vi "BuildCustomDashBoardData.vi"   [LabVIEW 2013]
doc: "This VI builds data and sends it back to the dashboard PC program. By default it sends back the raw values for the first analog, digital, and solenoid module. Modify it to send back the data you want to view. Consider adding higher level data to the Dashboard Datatype.ctl and to this VI. Then update the Dashboard to display the data however you like.\n\nThis software is licensed. Open the labview\\readme\\WPI Robotics Library Open Source License.txt file for more information."
uses:
  <vilib>/Rock Robotics/WPI/DriverStation/WPI_DriverStationDigitalData.ctl
  typedefs/Dashboard Datatype.ctl
  typedefs/DashboardEnable.ctl
  typedefs/custom dash data.ctl
  typedefs/subStates.ctl
  typedefs/vision data.ctl
  <vilib>/Rock Robotics/WPI/Joystick/WPI_JoystickButtonState.ctl
  typedefs/fg_typedef.ctl
  <vilib>/Rock Robotics/SystemInterfaces/System/FPGA_SystemGet.vi
  <vilib>/Rock Robotics/WPI/Joystick/WPI_JoystickGetSetRefNum.vi
  <vilib>/NI_Real-Time Target Support.lvlib
types:
  T1 = typedef "custom dash data.ctl" = cluster{"Motors":cluster{"Pickup Motor":dbl, "Pickup Belt":dbl, "Pickup Distance ":dbl, "Pickup Rate":dbl, "Right Motor":dbl, "Left Motor":dbl}, "substates":cluster{"Latch":T2, "Pickup Arm":T2, "Belts":T2, "Shooter":T2, "Drive":T2}, "Safeties":cluster{"Arm Safety":bool, "Arm Limit":bool}, "Performance":cluster{"CPU Usage":dbl, "Vision mSPI":u32, "Main mSPI":u32}, "Data":T3, "Joysticks":cluster{"J1 Axes":cluster{"axis 1 (x)":dbl, "axis 2 (y)":dbl, "axis 3 (throttle)":dbl, "axis 4":dbl, "axis 5":dbl, "axis 6":dbl}, "J1 Buttons":T4, "J2 Axes":cluster{"axis 1 (x)":dbl, "axis 2 (y)":dbl, "axis 3 (throttle)":dbl, "axis 4":dbl, "axis 5":dbl, "axis 6":dbl}, "J2 Buttons":T4, "J3 Axes":cluster{"axis 1 (x)":dbl, "axis 2 (y)":dbl, "axis 3 (throttle)":dbl, "axis 4":dbl, "axis 5":dbl, "axis 6":dbl}, "J3 Buttons":T4}, "SubSystem Manager":cluster{"Ball State Read":enum16{"no ball", "holding", "loaded"}, "Picked Up":bool, "Loaded":bool, "Shooter Cocked":bool, "Arm Ready":bool}, "Vision Enabled?":bool}
  T2 = typedef "subStates.ctl" = enum16{"null", "wait", "driver control", "auto", "manual override", "hold position", "rotate", "pickup", "pass", "load", "goto shoot", "shoot", "cancel", "end"}
  T3 = typedef "vision data.ctl" = cluster{"x":dbl, "y":dbl, "area":dbl, "width":dbl, "height":dbl, "Hot Goal Present?":bool, "distance":dbl}
  T4 = typedef "WPI_JoystickButtonState.ctl" = cluster{"Button 1":bool, "Button 2":bool, "Button 3":bool, "Button 4":bool, "Button 5":bool, "Button 6":bool, "Button 7":bool, "Button 8":bool, "Button 9":bool, "Button 10":bool, "Button 11":bool, "Button 12":bool}
  T5 = typedef "DashboardEnable.ctl" = cluster{"Analog Module 1":bool[], "Analog Module 2":bool[], "Digital Module 1":bool, "Digital Module 2":bool, "Solenoid Module":bool}
  T6 = typedef "Dashboard Datatype.ctl" = cluster{cluster{"AnalogModule[0]":cluster{"Channel[0]":sgl, "Channel[1]":sgl, "Channel[2]":sgl, "Channel[3]":sgl, "Channel[4]":sgl, "Channel[5]":sgl, "Channel[6]":sgl, "Channel[7]":sgl}, "AnalogModule[1]":cluster{"Channel[0]":sgl, "Channel[1]":sgl, "Channel[2]":sgl, "Channel[3]":sgl, "Channel[4]":sgl, "Channel[5]":sgl, "Channel[6]":sgl, "Channel[7]":sgl}}, cluster{"DigitalModule[0]":T7, "DigitalModule[1]":T7}, "Solenoid":u8}
  T7 = typedef "WPI_DriverStationDigitalData.ctl" = cluster{"Relay Fwd":u8, "Relay Rev":u8, "GPIO":u16, "GPIO_OE":u16, "PWM":cluster{"PWM[0]":u8, "PWM[1]":u8, "PWM[2]":u8, "PWM[3]":u8, "PWM[4]":u8, "PWM[5]":u8, "PWM[6]":u8, "PWM[7]":u8, "PWM[8]":u8, "PWM[9]":u8}}
  T8 = typedef "fg_typedef.ctl" = enum16{"Get", "Set"}
  T9 = cluster{"AnalogModule[0]":cluster{"Channel[0]":sgl, "Channel[1]":sgl, "Channel[2]":sgl, "Channel[3]":sgl, "Channel[4]":sgl, "Channel[5]":sgl, "Channel[6]":sgl, "Channel[7]":sgl}, "AnalogModule[1]":cluster{"Channel[0]":sgl, "Channel[1]":sgl, "Channel[2]":sgl, "Channel[3]":sgl, "Channel[4]":sgl, "Channel[5]":sgl, "Channel[6]":sgl, "Channel[7]":sgl}}
  T10 = cluster{"DigitalModule[0]":T7, "DigitalModule[1]":T7}
  T11 = cluster{"Channel[0]":sgl, "Channel[1]":sgl, "Channel[2]":sgl, "Channel[3]":sgl, "Channel[4]":sgl, "Channel[5]":sgl, "Channel[6]":sgl, "Channel[7]":sgl}[]
  T12 = cluster{"Channel[0]":sgl, "Channel[1]":sgl, "Channel[2]":sgl, "Channel[3]":sgl, "Channel[4]":sgl, "Channel[5]":sgl, "Channel[6]":sgl, "Channel[7]":sgl}
  T13 = cluster{"AnalogModule[0][0]":sgl, "AnalogModule[0][1]":sgl, "AnalogModule[0][2]":sgl, "AnalogModule[0][3]":sgl, "AnalogModule[0][4]":sgl, "AnalogModule[0][5]":sgl, "AnalogModule[0][6]":sgl, "AnalogModule[0][7]":sgl}
  T14 = cluster{"[0]":cluster{"Channel[0]":sgl, "Channel[1]":sgl, "Channel[2]":sgl, "Channel[3]":sgl, "Channel[4]":sgl, "Channel[5]":sgl, "Channel[6]":sgl, "Channel[7]":sgl}, "[1]":cluster{"Channel[0]":sgl, "Channel[1]":sgl, "Channel[2]":sgl, "Channel[3]":sgl, "Channel[4]":sgl, "Channel[5]":sgl, "Channel[6]":sgl, "Channel[7]":sgl}}
  T15 = typedef "FPGA_DIODevRef.ctl" = cluster{"DevStatus":errorcluster, "Module":T16}
  T16 = typedef "FPGA_TypedefDigitalModule.ctl" = enum16{"Digital Module 1", "Digital Module 2"}
  T17 = cluster{"[0]":u8, "[1]":u8, "[2]":u8, "[3]":u8, "[4]":u8, "[5]":u8, "[6]":u8, "[7]":u8, "[8]":u8, "[9]":u8}
  T18 = typedef "FPGA_SolenoidDevRef.ctl" = cluster{"DevStatus":errorcluster, "Module":T19}
  T19 = typedef "FPGA_TypedefSolenoidModule.ctl" = enum16{"Solenoid Module 1", "Solenoid Module 2"}
  T20 = cluster{"Pickup Motor":dbl, "Pickup Belt":dbl, "Pickup Distance ":dbl, "Pickup Rate":dbl, "Right Motor":dbl, "Left Motor":dbl}
  T21 = cluster{"CPU Usage":dbl, "Vision mSPI":u32, "Main mSPI":u32}
  T22 = typedef "WPI_EncoderDevRef.ctl" = cluster{"DevStatus":errorcluster, "EncoderIndex":T23, "CounterIndex":T24, "DistancePerCount":dbl, "Decoding Type":T25}
  T23 = typedef "FPGA_EncoderIdx.ctl" = enum8{"Enc 0", "Enc 1", "Enc 2", "Enc 3", "Invalid"}
  T24 = typedef "FPGA_CounterCtrSystemIndex.ctl" = enum8{"Ctr 0", "Ctr 1", "Ctr 2", "Ctr 3", "Ctr 4", "Ctr 5", "Ctr 6", "Ctr 7", "Invalid"}
  T25 = typedef "WPI_EncoderType.ctl" = enum16{"1x", "2x", "4x"}
  T26 = typedef "WPI_MotorControlDeviceRef.ctl" = cluster{"DeviceStatus":errorcluster, "Type":enum16{"PWM", "CAN"}, "PWM":cluster{"Digital Module":T16, "PWM Channel":T27, "DeadBand":T28}, "CAN":cluster{"Device Number":u8, "Control Mode":T29, "Semaphore":T30, "Max Vout":dbl}, "Invert":bool, "TransformRef":T31, "InvTransformRef":T31}
  T27 = typedef "FPGA_DIOPWMChannel.ctl" = enum8{"PWM 1", "PWM 2", "PWM 3", "PWM 4", "PWM 5", "PWM 6", "PWM 7", "PWM 8", "PWM 9", "PWM 10", "Invalid"}
  T28 = typedef "WPI_PWMDeadband.ctl" = cluster{"Name":string, "maxPositivePwm":i32, "minPositivePwm":i32, "centerPwm":i32, "maxNegativePwm":i32, "minNegativePwm":i32, "angularRange":u16}
  T29 = typedef "WPI_CANJaguar_ControlMode.ctl" = enum8{"Percent VBus", "Current", "Speed", "Position", "Voltage"}
  T30 = typedef "Semaphore RefNum" = refnum<k1>
  T31 = typedef "WPI_PWMTransform_ConPane.ctl" = refnum<vi>
  T32 = typedef "NI_Real-Time Target Support.lvlib/RT CPU Load.ctl" = cluster{"Total (%)":dbl, "Time Critical (%)":dbl, "Timed Structures (%)":dbl, "High (%)":dbl, "Above Normal (%)":dbl, "Normal (%)":dbl, "Background (%)":dbl, "Idle (%)":dbl, "ISR (%)":dbl}
  T33 = cluster{"Vision mSPI":u32, "Main mSPI":u32, "Dash mSPI":u32}
  T34 = cluster{"Ball State Read":enum16{"no ball", "holding", "loaded"}, "Picked Up":bool, "Loaded":bool, "Shooter Cocked":bool, "Arm Ready":bool}
  T35 = typedef "WPI_JoystickDevRef.ctl" = cluster{"Device":T36}
  T36 = typedef "WPI_JoystickDeviceEnum.ctl" = enum16{"USB 1", "USB 2", "USB 3", "USB 4", "Kinect 1", "Kinect 2"}
  T37 = cluster{"axis 1 (x)":dbl, "axis 2 (y)":dbl, "axis 3 (throttle)":dbl, "axis 4":dbl, "axis 5":dbl, "axis 6":dbl}
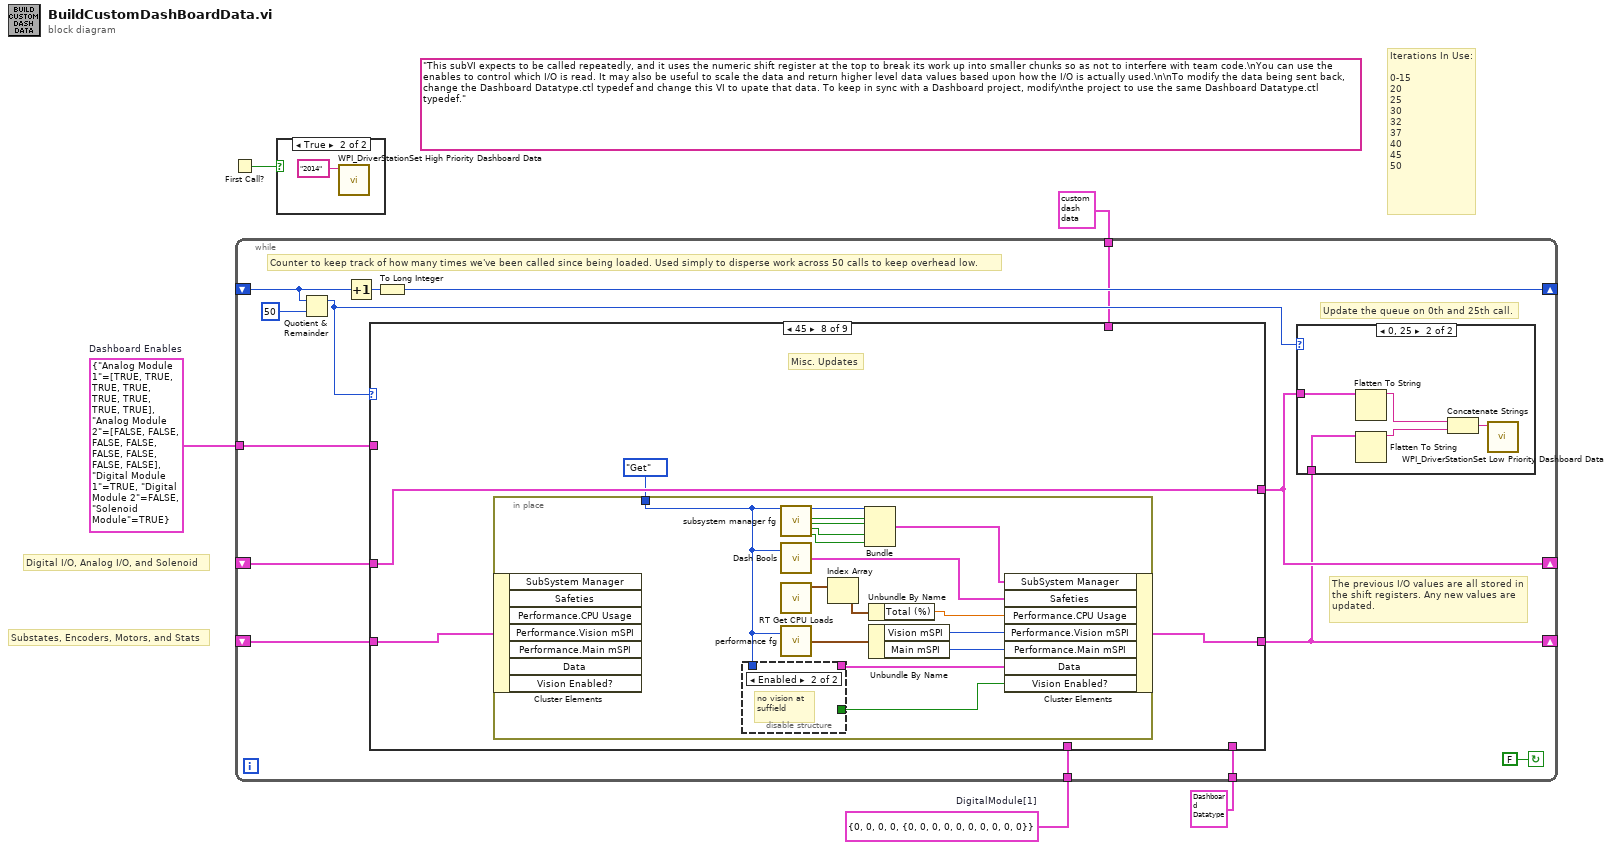
[diagram p0: block diagram]
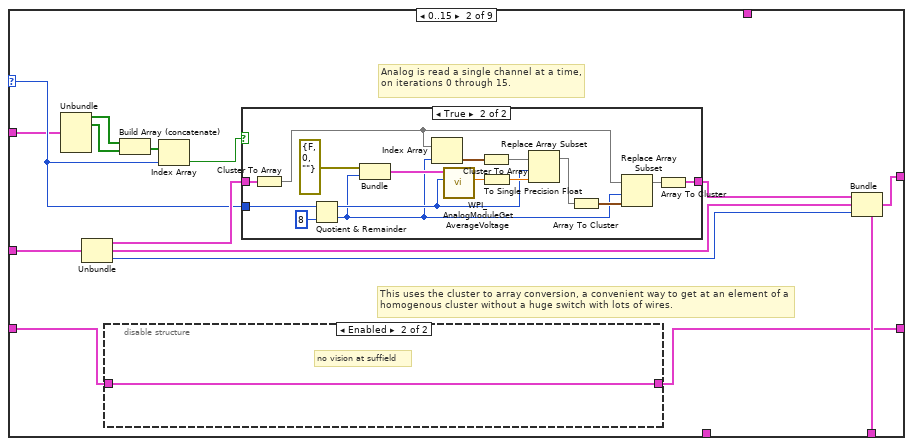
[diagram p5: hidden frame]
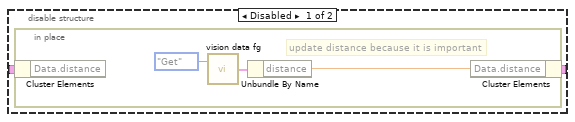
[diagram p6: hidden frame]
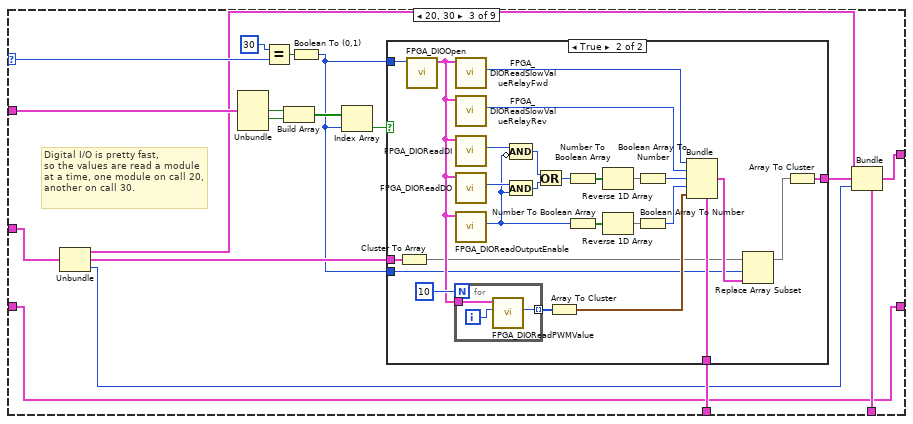
[diagram p8: hidden frame]
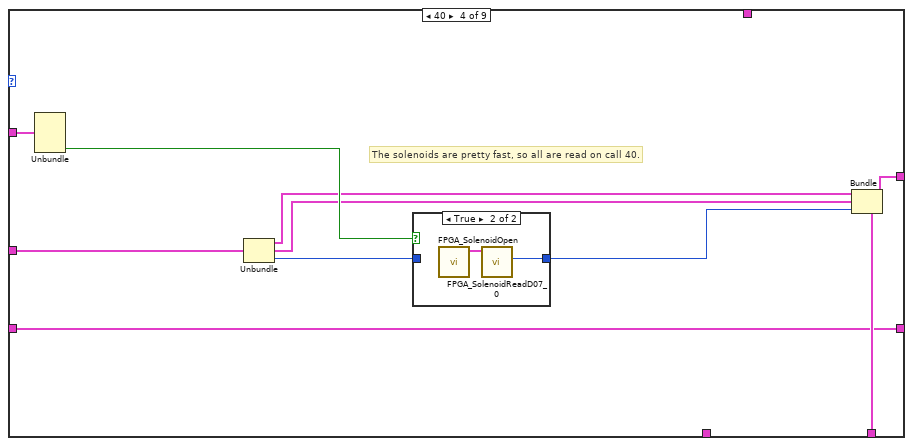
[diagram p10: hidden frame]
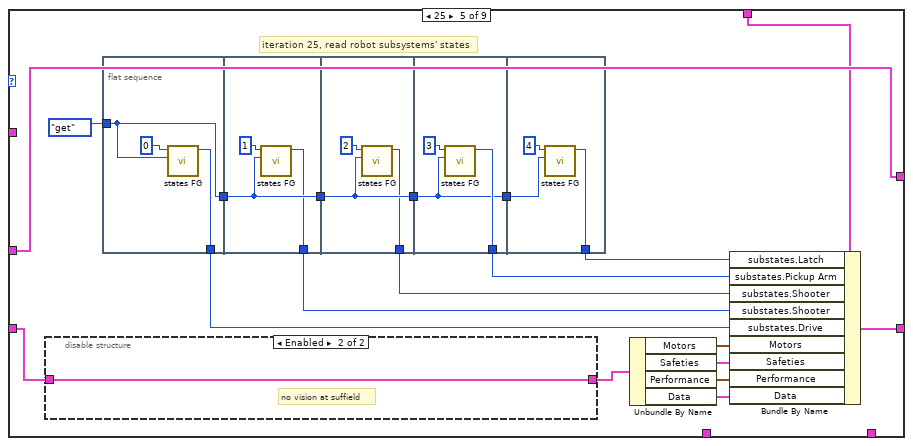
[diagram p12: hidden frame]
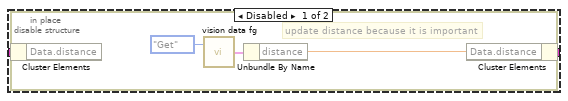
[diagram p13: hidden frame]
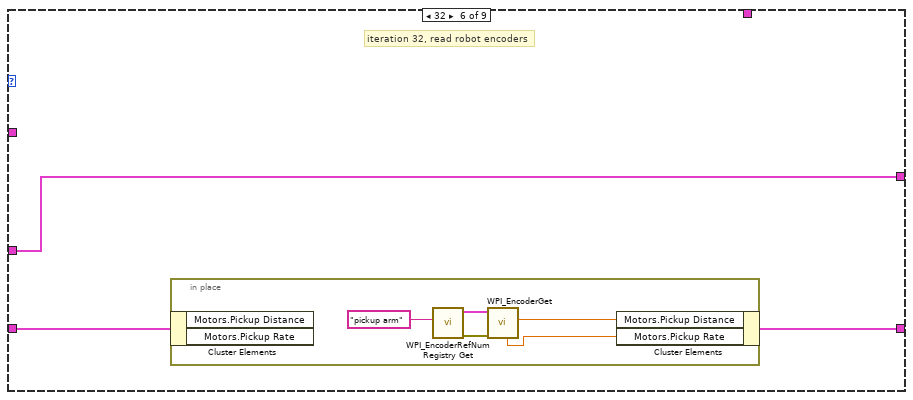
[diagram p14: hidden frame]
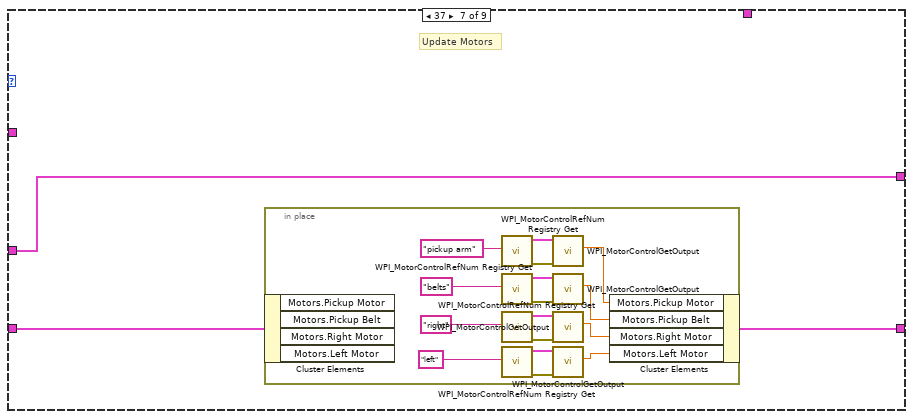
[diagram p15: hidden frame]
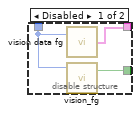
[diagram p16: hidden frame]
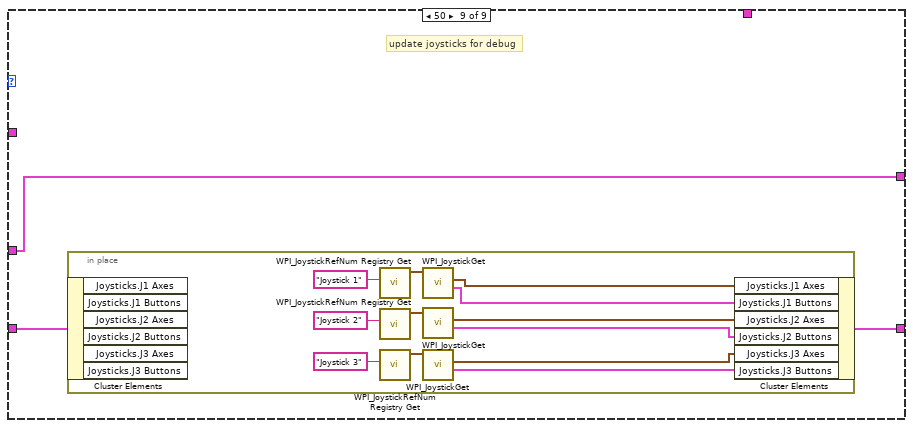
[diagram p17: hidden frame]
diagram:
  w5 = T5 {"Analog Module 1"=[TRUE, TRUE, TRUE, TRUE, TRUE, TRUE, TRUE, TRUE], "Analog Module 2"=[FALSE, FALSE, FALSE, FALSE, FALSE, FALSE, FALSE, FALSE], "Digital Module 1"=TRUE, "Digital Module 2"=FALSE, "Solenoid Module"=TRUE}  # Dashboard Enables
  (unwired) "This subVI expects to be called repeatedly, and it uses the numeric shift register at the top to break its work up into smaller chunks so as not to interfere with team code.\nYou can use the enables to control which I/O is read. It may also be useful to scale the data and return higher level data values based upon how the I/O is actually used.\n\nTo modify the data being sent back, change the Dashboard Datatype.ctl typedef and change this VI to upate that data. To keep in sync with a Dashboard project, modify\nthe project to use the same Dashboard Datatype.ctl typedef."
  w4 = T7 {"Relay Fwd"=0, "Relay Rev"=0, "GPIO"=0, "GPIO_OE"=0, "PWM"={"PWM[0]"=0, "PWM[1]"=0, "PWM[2]"=0, "PWM[3]"=0, "PWM[4]"=0, "PWM[5]"=0, "PWM[6]"=0, "PWM[7]"=0, "PWM[8]"=0, "PWM[9]"=0}}  # DigitalModule[1]
  # "Iterations In Use:\n\n0-15\n20\n25\n30\n32\n37\n40\n45\n50"
  # "Substates, Encoders, Motors, and Stats"
  # "Digital I/O, Analog I/O, and Solenoid"
  n1 = First Call?() -> (First Call?: T/F=w3:bool)
  n2 = while {
    shift-right: [w12] -> _
    shift-left: _ -> [w14]
    shift-right: [w9] -> _
    shift-left: _ -> [w17]
    tunnel: w4 -> [w16]
    tunnel: T6 {{"AnalogModule[0]"={"Channel[0]"=0.0, "Channel[1]"=0.0, "Channel[2]"=0.0, "Channel[3]"=0.0, "Channel[4]"=0.0, "Channel[5]"=0.0, "Channel[6]"=0.0, "Channel[7]"=0.0}, "AnalogModule[1]"={"Channel[0]"=0.0, "Channel[1]"=0.0, "Channel[2]"=0.0, "Channel[3]"=0.0, "Channel[4]"=0.0, "Channel[5]"=0.0, "Channel[6]"=0.0, "Channel[7]"=0.0}}, {"DigitalModule[0]"={"Relay Fwd"=0, "Relay Rev"=0, "GPIO"=0, "GPIO_OE"=0, "PWM"={"PWM[0]"=0, "PWM[1]"=0, "PWM[2]"=0, "PWM[3]"=0, "PWM[4]"=0, "PWM[5]"=0, "PWM[6]"=0, "PWM[7]"=0, "PWM[8]"=0, "PWM[9]"=0}}, "DigitalModule[1]"={"Relay Fwd"=0, "Relay Rev"=0, "GPIO"=0, "GPIO_OE"=0, "PWM"={"PWM[0]"=0, "PWM[1]"=0, "PWM[2]"=0, "PWM[3]"=0, "PWM[4]"=0, "PWM[5]"=0, "PWM[6]"=0, "PWM[7]"=0, "PWM[8]"=0, "PWM[9]"=0}}}, "Solenoid"=0} ("Dashboard Data") -> [w11]
    tunnel: w5 -> [w10]
    shift-right: [w6] -> _
    shift-left: _ -> [w7]
    tunnel: T1 {"Motors"={"Pickup Motor"=0.0, "Pickup Belt"=0.0, "Pickup Distance "=0.0, "Pickup Rate"=0.0, "Right Motor"=0.0, "Left Motor"=0.0}, "substates"={"Latch"=enum."null", "Pickup Arm"=enum."null", "Belts"=enum."null", "Shooter"=enum."null", "Drive"=enum."null"}, "Safeties"={"Arm Safety"=FALSE, "Arm Limit"=FALSE}, "Performance"={"CPU Usage"=0.0, "Vision mSPI"=0, "Main mSPI"=0}, "Data"={"x"=0.0, "y"=0.0, "area"=0.0, "width"=0.0, "height"=0.0, "Hot Goal Present?"=FALSE, "distance"=0.0}, "Joysticks"={"J1 Axes"={"axis 1 (x)"=0.0, "axis 2 (y)"=0.0, "axis 3 (throttle)"=0.0, "axis 4"=0.0, "axis 5"=0.0, "axis 6"=0.0}, "J1 Buttons"={"Button 1"=FALSE, "Button 2"=FALSE, "Button 3"=FALSE, "Button 4"=FALSE, "Button 5"=FALSE, "Button 6"=FALSE, "Button 7"=FALSE, "Button 8"=FALSE, "Button 9"=FALSE, "Button 10"=FALSE, "Button 11"=FALSE, "Button 12"=FALSE}, "J2 Axes"={"axis 1 (x)"=0.0, "axis 2 (y)"=0.0, "axis 3 (throttle)"=0.0, "axis 4"=0.0, "axis 5"=0.0, "axis 6"=0.0}, "J2 Buttons"={"Button 1"=FALSE, "Button 2"=FALSE, "Button 3"=FALSE, "Button 4"=FALSE, "Button 5"=FALSE, "Button 6"=FALSE, "Button 7"=FALSE, "Button 8"=FALSE, "Button 9"=FALSE, "Button 10"=FALSE, "Button 11"=FALSE, "Button 12"=FALSE}, "J3 Axes"={"axis 1 (x)"=0.0, "axis 2 (y)"=0.0, "axis 3 (throttle)"=0.0, "axis 4"=0.0, "axis 5"=0.0, "axis 6"=0.0}, "J3 Buttons"={"Button 1"=FALSE, "Button 2"=FALSE, "Button 3"=FALSE, "Button 4"=FALSE, "Button 5"=FALSE, "Button 6"=FALSE, "Button 7"=FALSE, "Button 8"=FALSE, "Button 9"=FALSE, "Button 10"=FALSE, "Button 11"=FALSE, "Button 12"=FALSE}}, "SubSystem Manager"={"Ball State Read"=enum."no ball", "Picked Up"=FALSE, "Loaded"=FALSE, "Shooter Cocked"=FALSE, "Arm Ready"=FALSE}, "Vision Enabled?"=FALSE} ("Custom Dash Data") -> [w8]
    stop <- FALSE continue-if-true
    # "Counter to keep track of how many times we've been called since being loaded. Used simply to disperse work across 50 calls to keep overhead low."
    # "Update the queue on 0th and 25th call."
    # "The previous I/O values are all stored in\nthe shift registers. Any new values are\nupdated."
    n3 = Quotient & Remainder(x=w14, y=50) -> (x-y*floor(x/y)=w13:i32)  [unwired: 1 out]
    n4 = Increment(x=w14) -> (x+1=w19:i32)
    n5 = case shown="45" w13 {
      selector: w13 -> [_ w36 w78 _ _ _ _ _ _]
      tunnel: [w26 w32 w69 w119 w134 w167 w176 w195 w218] -> w9
      tunnel: w17 -> [w26 w31 w71 w121 w134 w167 w176 w195 w218]
      tunnel: w16 -> [_ _ w82 _ _ _ _ _ _]
      tunnel: w11 -> [_ w38 w70 w118 _ _ _ _ _]
      tunnel: w10 -> [_ w35 w76 w122 _ _ _ _ _]
      tunnel: w8 -> [_ _ _ _ w132 _ _ _ _]
      tunnel: [w25 w27 w67 w115 w133 w168 w175 w196 w216] -> w6
      tunnel: w7 -> [w25 w28 w67 w115 w128 w166 w174 w194 w217]
      frame Default {
        # "Don't update any I/O"
      }
      frame 0..15 {
        # "This uses the cluster to array conversion, a convenient way to get at an element of a\nhomogenous cluster without a huge switch with lots of wires."
        # "Analog is read a single channel at a time,\non iterations 0 through 15."
        n6 = Unbundle(w35) -> ("Analog Module 1"=w34:bool[], "Analog Module 2"=w33:bool[])  [unwired: 3 out]
        n7 = Unbundle(w31) -> (w37:T9, w30:T10, "Solenoid"=w29:u8)
        n8 = disable-structure shown="Enabled" {
          disable-tunnel: w28 -> [w43 w47]
          disable-tunnel: [w42 w47] -> w27
          frame Disabled {
            n9 = in-place {
              # "update distance because it is important"
              n10 = in-place-cluster #1(w43) -> ()  [unwired: 1 out]
              n11 = call "vision data fg.vi"("Menu"=fg_typedef."Get") -> ("Output"=w45:T3)  [unwired: 1 in]
              n12 = Unbundle By Name(w45) -> ("distance"=w44:dbl)
              n13 = in-place-cluster #1("Data.distance"=w44) -> (w42:T1)
            }
          }
          frame Enabled {
            # "no vision at suffield"
          }
        }
        n14 = Build Array (concatenate)(w34, w33) -> (w40:bool[])
        n15 = Index Array(array=w40, index=w36) -> (element=w41:bool)
        n16 = case shown="True" w41 {
          tunnel: w36 -> [_ w55]
          tunnel: [w48 w52] -> w39
          tunnel: w37 -> [w48 w51]
          frame False {
          }
          frame True {
            n17 = Cluster To Array(cluster=w51) -> (array=w50:T11)
            n18 = Quotient & Remainder(x=w55, y=8) -> (x-y*floor(x/y)=w54:i32, floor(x/y)=w49:i32)
            n19 = Bundle("DevStatus"=errorcluster {"status"=FALSE, "code"=0, "source"=""}, w49) -> (w63:cluster{"DevStatus":errorcluster, i32})  [unwired: 1 out]
            n20 = Index Array(array=w50, index=w49) -> (element=w57:T12)
            n21 = call <vilib>:"WPI_AnalogModuleGetAverageVoltage.vi"("Channel"=w54, "AnalogModuleDevStatus"=w63) -> ("Average Voltage"=w60:dbl)  [unwired: 1 in, 8 out]
            n22 = Cluster To Array(cluster=w57) -> (array=w56:sgl[])
            n23 = To Single Precision Float(number=w60) -> (single precision float=w59:sgl)
            n24 = Replace Array Subset(array=w56, new element=w59, index=w54) -> (w58:sgl[])
            n25 = Array To Cluster(array=w58) -> (cluster=w62:T13)
            n26 = Replace Array Subset(array=w50, new element=w62, index=w49) -> (w53:T11)
            n27 = Array To Cluster(array=w53) -> (cluster=w52:T14)
          }
        }
        n28 = Bundle(cluster=w38, w39, w30, "Solenoid"=w29) -> (w32:T6)
      }
      frame 20, 30 {
        # "Digital I/O is pretty fast,\nso the values are read a module\nat a time, one module on call 20,\nanother on call 30."
        n29 = Unbundle(w71) -> (w66:T9, w73:T10, "Solenoid"=w65:u8)
        n30 = Unbundle(w76) -> ("Digital Module 1"=w75:bool, "Digital Module 2"=w74:bool)  [unwired: 3 out]
        n31 = Equal?(x=30, y=w78) -> (x = y?=w80:bool)
        n32 = Build Array(w75, w74) -> (w77:bool[])
        n33 = Boolean To (0,1)(Boolean=w80) -> (0, 1=w68:i16)
        n34 = Index Array(array=w77, index=w68) -> (element=w79:bool)
        n35 = case shown="True" w79 {
          tunnel: w82 -> [_ w91]
          tunnel: [w83 w84] -> w72
          tunnel: w68 -> [_ w89]
          tunnel: w68 -> [_ w88]
          tunnel: w73 -> [w83 w87]
          frame False {
          }
          frame True {
            n36 = Cluster To Array(cluster=w87) -> (array=w86:T7[])
            n37 = call <vilib>:"FPGA_DIOOpen.vi"("Module (Module 1)"=w89) -> ("DIODeviceRef"=w107:T15)  [unwired: 1 in, 9 out]
            n38 = for {
              N: 10 -> [_]
              tunnel: w107 -> [w112]
              tunnel: [w110] -> w108 mode=indexing
              i -> [w111]
              n39 = call <vilib>:"FPGA_DIOReadPWMValue.vi"("PWMChannel"=w111, "DIODeviceRef In"=w112) -> ("PWMValue"=w110:u8)  [unwired: 1 in, 8 out]
            }
            n40 = call <vilib>:"FPGA_DIOReadSlowValueRelayFwd.vi"("DIODeviceRef In"=w107) -> ("Relay Forward"=w100:u8)  [unwired: 1 in, 9 out]
            n41 = call <vilib>:"FPGA_DIOReadSlowValueRelayRev.vi"("DIODeviceRef In"=w107) -> ("Relay Reverse"=w101:u8)  [unwired: 1 in, 9 out]
            n42 = call <vilib>:"FPGA_DIOReadDI.vi"("DIODeviceRef In"=w107) -> ("DI"=w105:u16)  [unwired: 1 in, 9 out]
            n43 = call <vilib>:"FPGA_DIOReadDO.vi"("DIODeviceRef In"=w107) -> ("DO"=w104:u16)  [unwired: 1 in, 9 out]
            n44 = call <vilib>:"FPGA_DIOReadOutputEnable.vi"("DIODeviceRef In"=w107) -> ("OutputEnable"=w95:u16)  [unwired: 1 in, 9 out]
            n45 = And(x=w104, y=w95) -> (x .and. y?=w103:u16)
            n46 = Compound Arithmetic op=AND(w105, invert w95) -> (w102:u16)
            n47 = Or(x=w102, y=w103) -> (x .or. y?=w93:u16)
            n48 = Array To Cluster(array=w108) -> (cluster=w106:T17)
            n49 = Number To Boolean Array(number=w93) -> (Boolean array=w98:bool[])
            n50 = Number To Boolean Array(number=w95) -> (Boolean array=w97:bool[])
            n51 = Reverse 1D Array(array=w98) -> (reversed array=w99:bool[])
            n52 = Reverse 1D Array(array=w97) -> (reversed array=w96:bool[])
            n53 = Boolean Array To Number(Boolean array=w99) -> (number=w92:u32)
            n54 = Boolean Array To Number(Boolean array=w96) -> (number=w94:u32)
            n55 = Bundle(cluster=w91, "Relay Fwd"=w100, "Relay Rev"=w101, "GPIO"=w92, "GPIO_OE"=w94, "PWM"=w106) -> (w90:T7)
            n56 = Replace Array Subset(array=w86, new element=w90, index=w88) -> (w85:T7[])
            n57 = Array To Cluster(array=w85) -> (cluster=w84:cluster{"[0]":T7, "[1]":T7})
          }
        }
        n58 = Bundle(cluster=w70, w66, w72, "Solenoid"=w65) -> (w69:T6)
      }
      frame 40 {
        # "The solenoids are pretty fast, so all are read on call 40."
        n59 = Unbundle(w122) -> ("Solenoid Module"=w116:bool)  [unwired: 4 out]
        n60 = Unbundle(w121) -> (w114:T9, w113:T10, "Solenoid"=w120:u8)
        n61 = case shown="True" w116 {
          tunnel: [w123 w124] -> w117
          tunnel: w120 -> [w123 _]
          frame False {
          }
          frame True {
            n62 = call <vilib>:"FPGA_SolenoidOpen.vi"() -> ("SolenoidDevRef"=w125:T18)  [unwired: 2 in, 9 out]
            n63 = call <vilib>:"FPGA_SolenoidReadD07_0.vi"("SolenoidDevRef"=w125) -> ("DO7:0"=w124:u8)  [unwired: 1 in, 9 out]
          }
        }
        n64 = Bundle(cluster=w118, w114, w113, "Solenoid"=w117) -> (w119:T6)
      }
      frame 25 {
        # "iteration 25, read robot subsystems' states"
        n65 = disable-structure shown="Enabled" {
          disable-tunnel: w128 -> [w146 w150]
          disable-tunnel: [w145 w150] -> w127
          frame Disabled {
            n66 = in-place {
              # "update distance because it is important"
              n67 = in-place-cluster #2(w146) -> ()  [unwired: 1 out]
              n68 = call "vision data fg.vi"("Menu"=fg_typedef."Get") -> ("Output"=w148:T3)  [unwired: 1 in]
              n69 = Unbundle By Name(w148) -> ("distance"=w147:dbl)
              n70 = in-place-cluster #2("Data.distance"=w147) -> (w145:T1)
            }
          }
          frame Enabled {
            # "no vision at suffield"
          }
        }
        n71 = flat-sequence {
          tunnel: enum16{"set", "get"}."get" ("menu (get)") -> [w153]
          tunnel: [w153] -> w141
          tunnel: [w151] -> w135
          tunnel: [w156] -> w142
          tunnel: w141 -> [w156]
          tunnel: [w154] -> w136
          tunnel: [w159] -> w143
          tunnel: w142 -> [w159]
          tunnel: [w157] -> w137
          tunnel: w143 -> [w160]
          tunnel: [w161] -> w138
          tunnel: [w160] -> w140
          tunnel: w140 -> [w164]
          tunnel: [w163] -> w139
          frame #0 {
            n72 = call "states FG.vi"("menu (get)"=w153, "Loop ID"=0) -> ("subState out"=w151:T2)  [unwired: 6 in, 3 out]
          }
          frame #1 {
            n73 = call "states FG.vi"("menu (get)"=w156, "Loop ID"=1) -> ("subState out"=w154:T2)  [unwired: 6 in, 3 out]
          }
          frame #2 {
            n74 = call "states FG.vi"("menu (get)"=w159, "Loop ID"=2) -> ("subState out"=w157:T2)  [unwired: 6 in, 3 out]
          }
          frame #3 {
            n75 = call "states FG.vi"("menu (get)"=w160, "Loop ID"=3) -> ("subState out"=w161:T2)  [unwired: 6 in, 3 out]
          }
          frame #4 {
            n76 = call "states FG.vi"("menu (get)"=w164, "Loop ID"=4) -> ("subState out"=w163:T2)  [unwired: 6 in, 3 out]
          }
        }
        n77 = Unbundle By Name(w127) -> ("Motors"=w126:T20, "Safeties"=w131:cluster{"Arm Safety":bool, "Arm Limit":bool}, "Performance"=w130:T21, "Data"=w129:T3)
        n78 = Bundle By Name(cluster=w132, "substates.Latch"=w139, "substates.Pickup Arm"=w138, "substates.Shooter"=w137, "substates.Shooter"=w136, "substates.Drive"=w135, "Motors"=w126, "Safeties"=w131, "Performance"=w130, "Data"=w129) -> (w133:T1)
      }
      frame 32 {
        # "iteration 32, read robot encoders"
        n79 = in-place {
          n80 = in-place-cluster #3(w166) -> ()  [unwired: 2 out]
          n81 = call <vilib>:"WPI_EncoderRefNum Registry Get.vi"("refnum name"="pickup arm") -> ("error out"=w172:errorcluster, "EncoderDevRef"=w173:T22)  [unwired: 9 in]
          n82 = call <vilib>:"WPI_EncoderGet.vi"("error in (no error)"=w172, "EncoderDevRef"=w173) -> ("Distance"=w170:dbl, "Rate"=w169:dbl)  [unwired: 4 in, 4 out]
          n83 = in-place-cluster #3("Motors.Pickup Distance"=w170, "Motors.Pickup Rate"=w169) -> (w168:T1)
        }
      }
      frame 37 {
        # "Update Motors"
        n84 = in-place {
          n85 = in-place-cluster #4(w174) -> ()  [unwired: 4 out]
          n86 = call <vilib>:"WPI_MotorControlRefNum Registry Get.vi"("refnum name"="pickup arm") -> ("error out"=w185:errorcluster, "MotorControlDevRef"=w189:T26)  [unwired: 9 in]
          n87 = call <vilib>:"WPI_MotorControlRefNum Registry Get.vi"("refnum name"="belts") -> ("error out"=w186:errorcluster, "MotorControlDevRef"=w192:T26)  [unwired: 9 in]
          n88 = call <vilib>:"WPI_MotorControlRefNum Registry Get.vi"("refnum name"="right") -> ("error out"=w184:errorcluster, "MotorControlDevRef"=w182:T26)  [unwired: 9 in]
          n89 = call <vilib>:"WPI_MotorControlRefNum Registry Get.vi"("refnum name"="left") -> ("error out"=w179:errorcluster, "MotorControlDevRef"=w181:T26)  [unwired: 9 in]
          n90 = call <vilib>:"WPI_MotorControlGetOutput.vi"("error in (no error)"=w185, "MotorControlDevRef"=w189) -> ("Output"=w188:dbl)  [unwired: 7 in, 2 out]
          n91 = call <vilib>:"WPI_MotorControlGetOutput.vi"("error in (no error)"=w186, "MotorControlDevRef"=w192) -> ("Output"=w187:dbl)  [unwired: 7 in, 2 out]
          n92 = call <vilib>:"WPI_MotorControlGetOutput.vi"("error in (no error)"=w184, "MotorControlDevRef"=w182) -> ("Output"=w177:dbl)  [unwired: 7 in, 2 out]
          n93 = call <vilib>:"WPI_MotorControlGetOutput.vi"("error in (no error)"=w179, "MotorControlDevRef"=w181) -> ("Output"=w178:dbl)  [unwired: 7 in, 2 out]
          n94 = in-place-cluster #4("Motors.Pickup Motor"=w188, "Motors.Pickup Belt"=w187, "Motors.Right Motor"=w177, "Motors.Left Motor"=w178) -> (w175:T1)
        }
      }
      frame 45 {
        # "Misc. Updates"
        n95 = in-place {
          in-place-border: fg_typedef."Get" ("Menu (Get)") -> [w198]
          n96 = in-place-cluster #5(w194) -> ()  [unwired: 7 out]
          n97 = disable-structure shown="Enabled" {
            disable-tunnel: [w215 _] -> w205
            disable-tunnel: w198 -> [w214 _]
            disable-tunnel: [w213 _] -> w197
            frame Disabled {
              n98 = call "vision data fg.vi"("Menu"=w214) -> ("Output"=w215:T3)  [unwired: 1 in]
              n99 = call "vision_fg.vi"("Menu"=w214) -> ("Enabled?"=w213:bool)  [unwired: 2 in, 1 out]
            }
            frame Enabled {
              # "no vision at\nsuffield"
            }
          }
          n100 = call "subsystem manager fg.vi"("Menu"=w198) -> ("Ball State Read"=w204:enum16{"no ball", "holding", "loaded"}, "Picked Up"=w203:bool, "Loaded"=w202:bool, "Shooter Cocked"=w201:bool, "Arm Ready"=w200:bool)  [unwired: 14 in]
          n101 = call "Dash Bools.vi"("Menu"=w198) -> ("Output"=w206:cluster{"Arm Safety":bool, "Arm Limit":bool})  [unwired: 1 in]
          n102 = call <vilib>:"RT Get CPU Loads.vi"() -> ("CPU loads"=w211:T32[])  [unwired: 10 in, 1 out]
          n103 = call "performance fg.vi"("Menu"=w198) -> ("Output"=w207:T33)  [unwired: 1 in]
          n104 = Index Array(array=w211) -> (element=w212:T32)  [unwired: 1 in]
          n105 = Bundle("Ball State Read"=w204, "Picked Up"=w203, "Loaded"=w202, "Shooter Cocked"=w201, "Arm Ready"=w200) -> (w199:T34)  [unwired: 1 in]
          n106 = Unbundle By Name(w212) -> ("Total (%)"=w210:dbl)
          n107 = Unbundle By Name(w207) -> ("Vision mSPI"=w209:u32, "Main mSPI"=w208:u32)
          n108 = in-place-cluster #5("SubSystem Manager"=w199, "Safeties"=w206, "Performance.CPU Usage"=w210, "Performance.Vision mSPI"=w209, "Performance.Main mSPI"=w208, "Data"=w205, "Vision Enabled?"=w197) -> (w196:T1)
        }
      }
      frame 50 {
        # "update joysticks for debug"
        n109 = in-place {
          n110 = in-place-cluster #6(w217) -> ()  [unwired: 6 out]
          n111 = call <vilib>:"WPI_JoystickRefNum Registry Get.vi"("refnum name"="Joystick 1") -> ("JoystickDevRef"=w227:T35)  [unwired: 9 in, 1 out]
          n112 = call <vilib>:"WPI_JoystickRefNum Registry Get.vi"("refnum name"="Joystick 2") -> ("JoystickDevRef"=w226:T35)  [unwired: 9 in, 1 out]
          n113 = call <vilib>:"WPI_JoystickRefNum Registry Get.vi"("refnum name"="Joystick 3") -> ("JoystickDevRef"=w225:T35)  [unwired: 9 in, 1 out]
          n114 = call <vilib>:"WPI_JoystickGet.vi"("JoystickDevRef"=w227) -> ("Buttons"=w220:T4, "Axes"=w219:T37)  [unwired: 4 in, 1 out]
          n115 = call <vilib>:"WPI_JoystickGet.vi"("JoystickDevRef"=w226) -> ("Buttons"=w222:T4, "Axes"=w221:T37)  [unwired: 4 in, 1 out]
          n116 = call <vilib>:"WPI_JoystickGet.vi"("JoystickDevRef"=w225) -> ("Buttons"=w223:T4, "Axes"=w224:T37)  [unwired: 4 in, 1 out]
          n117 = in-place-cluster #6("Joysticks.J1 Axes"=w219, "Joysticks.J1 Buttons"=w220, "Joysticks.J2 Axes"=w221, "Joysticks.J2 Buttons"=w222, "Joysticks.J3 Axes"=w224, "Joysticks.J3 Buttons"=w223) -> (w216:T1)
        }
      }
    }
    n118 = To Long Integer(number=w19) -> (32bit integer=w12:i32)
    n119 = case shown="0, 25" w13 {
      tunnel: w9 -> [_ w24]
      tunnel: w6 -> [_ w22]
      frame Default {
      }
      frame 0, 25 {
        n120 = Flatten To String(anything=w24) -> (data string=w23:string)  [unwired: 1 in, 4 out]
        n121 = Flatten To String(anything=w22) -> (data string=w20:string)  [unwired: 1 in, 4 out]
        n122 = Concatenate Strings(w23, w20) -> (w21:string)
        n123 = call <vilib>:"WPI_DriverStationSet Low Priority Dashboard Data.vi"("User Data"=w21) -> ()  [unwired: 1 in, 10 out]
      }
    }
  }
  n124 = case shown="True" w3 {
    frame False {
    }
    frame True {
      n125 = call <vilib>:"WPI_DriverStationSet High Priority Dashboard Data.vi"("User Data"="2014") -> ()  [unwired: 10 in, 1 out]
    }
  }
